vi "configuration UI.vi"() -> ()   [LabVIEW 2013, in "Modbus Module editor node.lvclass"]
doc: "Platypus Framework 1.0.1.65\nNI Systems Engineering - National Instruments"
uses:
  Modbus Module editor node.lvclass
  <vilib>/NI/Configuration Framework/Node/NodeRef.ctl
  <vilib>/NI/Configuration Framework/Node/NISE_CEF_Node.lvclass
  <vilib>/NI/AMC/Message Queue.ctl
  <vilib>/NI/AMC/Message.ctl
  <vilib>/NI/Tools/Keyed Array/KeyedArray.ctl
  <vilib>/NI/Configuration Framework/Node/UserEventRef.ctl
  <vilib>/NI/Configuration Framework/Controls/EventCluster.ctl
  <vilib>/NI/DCAF UI Toolkit/Controls/Configure.ctl
  <vilib>/NI/DCAF UI Toolkit/Controls/Add.ctl
  <vilib>/NI/DCAF UI Toolkit/Controls/Remove.ctl
  <vilib>/NI/DCAF UI Toolkit/Controls/Export.ctl
  module/configuration/modbus class.ctl
  <vilib>/NI/Configuration Framework/Node/NodeChangeEvent.ctl
  <vilib>/NI/DCAF/Tag Editor Core/control module/editor node/channel action event.ctl
  <vilib>/NI/DCAF/Tag Editor Core/control module/editor node/dialog output action.ctl
  <vilib>/NI/Tag Bus Module Framework/channel/TBM channel.lvclass
  <vilib>/NI/Tag Bus/tag/tag descriptor.lvclass
  <vilib>/NI/Configuration Framework/Node/CacheState.ctl
  <vilib>/NI/Configuration Framework/Node/StopEvent.ctl
  <vilib>/NI/Configuration Framework/Node/RefreshUIEvent.ctl
  <vilib>/Utility/miscctls.llb/LVRowAndColumnTypeDef.ctl
  <vilib>/NI/DCAF Table API/Listbox/Multi Column Listbox.lvclass
  <vilib>/NI/DCAF Table API/Table Manager/references.ctl
  <vilib>/NI/DCAF Table API/Listbox/Multi Column Listbox.lvclass/Multi Column Listbox.ctl
  <vilib>/NI/DCAF Table API/Table Manager/Table Manager.lvclass/Table Manager.ctl
  module/configuration/Modbus Module configuration.lvclass
  module/configuration/Modbus Module configuration.lvclass/Modbus Module configuration.ctl
  <vilib>/NI/DCAF/Tag Editor Core/Configuration Editor/Classes/Module editor node/module editor node.lvclass
  module/configuration/modbus mapping behavior.ctl
  module/configuration/Read port (502).vi
  module/configuration/Read baud rate.vi
  module/configuration/Read class.vi
  module/configuration/Read flow control (none).vi
  module/configuration/Read parity (even).vi
  module/configuration/Read serial type.vi
  module/configuration/Read unit ID.vi
  module/configuration/Read VISA resource name.vi
  module/configuration/Read IP address.vi
  module/configuration/Write port (502).vi
  module/configuration/Write baud rate.vi
  module/configuration/Write class.vi
  module/configuration/Write flow control (none).vi
  module/configuration/Write parity (even).vi
  module/configuration/Write serial type.vi
  module/configuration/Write unit ID.vi
  module/configuration/Write VISA resource name.vi
  module/configuration/Write IP address.vi
  module/configuration/Read modbus channels.vi
  <vilib>/NI/DCAF Table API/Listbox/Write Listbox.vi
  <vilib>/NI/DCAF Table API/Table Manager/Write Top VI.vi
  <vilib>/NI/DCAF/Tag Editor Core/Configuration Editor/Classes/Module editor node/Read Module Configuration.vi
  module/configuration/get wire mode.vi
  module/configuration/read force wire mode.vi
  module/configuration/set force wire mode.vi
  module/configuration/set wire mode.vi
  <vilib>/NI/Tag Bus Module Framework/module configuration/TBM module configuration.lvclass
  module/module channel/Modbus Module Channel.lvclass
  <vilib>/NI/Configuration Framework/NISE_CEF_TreeControl.lvlib
  <vilib>/NI/DCAF/Tag Editor Core/control module/editor node/control module editor.lvclass
  <vilib>/NI/Tools/Keyed Array/Tools_KeyedArray.lvlib
  <vilib>/NI/AMC/AMC.lvlib
  <vilib>/NI/DCAF Table API/Table Manager/Table Manager.lvclass
  <vilib>/NI/DCAF UI Toolkit/Controls/DCAF UI Elements.lvlib
panel:
  in  "refresh UI":T1
  in  "stop event":T2
  in  "cache state":T3
  in  "user event out":refnum<user-event>
  in  "node change":T4
  in  "Top Level Tab Control":enum32{"Registers", "Interface", "Export"}(tab)
  in  "settings":T5
  in  "channel":i32(listbox)=1
  in  "Add Button":T6
  in  "Remove Button":T7
  in  "remap":bool
  in  "Settings Tab Control":enum32{"TCP", "Serial"}(tab)
  in  "address":string
  in  "port (502)":u16=502
  in  "set wire mode?":bool
  in  "Wire Mode":T8(ring)
  in  "baud rate":u32
  in  "flow control (none)":u16
  in  "Serial Type":enum16{"RTU", "ASCII"}(ring)
  in  "VISA resource name":refnum<visa-resource-name>
  in  "Parity":enum16{"None", "Odd", "Even", "Mark", "Space"}(ring)
  in  "Unit ID":u8
  in  "Class":T9
  in  "export":T10
  in  "user event":T11
  in  "main queue":T12
  in  "node ref":T13
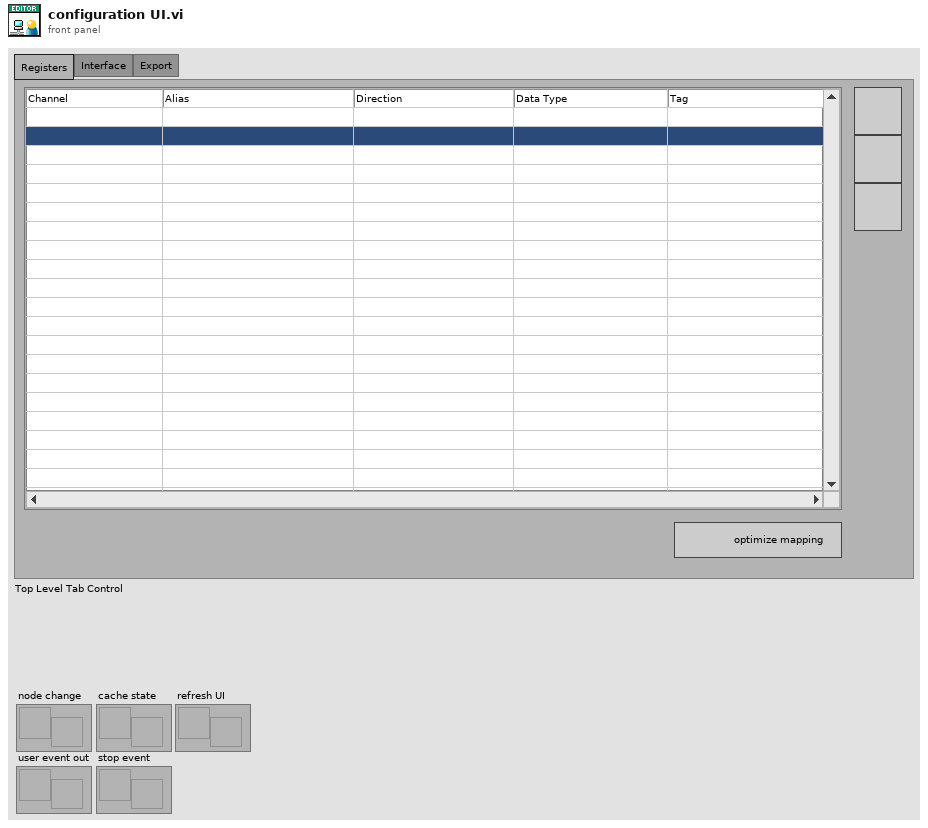
[diagram p1: front panel]
types:
  T1 = typedef "NISE_CEF_Node.lvclass/RefreshUIEvent.ctl" = refnum<user-event>
  T2 = typedef "NISE_CEF_Node.lvclass/StopEvent.ctl" = refnum<user-event>
  T3 = typedef "NISE_CEF_Node.lvclass/CacheState.ctl" = refnum<user-event>
  T4 = typedef "NISE_CEF_Node.lvclass/NodeChangeEvent.ctl" = refnum<user-event>
  T5 = typedef "DCAF UI Elements.lvlib/Configure.ctl" = bool
  T6 = typedef "DCAF UI Elements.lvlib/Add.ctl" = bool
  T7 = typedef "DCAF UI Elements.lvlib/Remove.ctl" = bool
  T8 = enum16{"Unknown", "RS485/Wire4", "RS485/Wire2-EchoDTR", "RS485/Wire2-CtrlDTR", "RS485/Wire2-Auto", "RS232/DTE", "RS232/DCE", "RS232/AUTO"}
  T9 = typedef "Modbus Module configuration.lvclass/modbus class.ctl" = enum16{"TCP master", "TCP slave", "serial master", "serial slave"}
  T10 = typedef "DCAF UI Elements.lvlib/Export.ctl" = bool
  T11 = typedef "NISE_CEF_Node.lvclass/UserEventRef.ctl" = refnum<user-event>
  T12 = typedef "AMC.lvlib/Message Queue.ctl" = refnum<queue>
  T13 = typedef "NISE_CEF_Node.lvclass/NodeRef.ctl" = refnum<data-value>
  T14 = typedef "Table Manager.lvlib/Table Manager.lvclass/references.ctl" = cluster{"stop event":T2, "refresh UI":T1, "cache state":T3, "node change":T4, "user event out":refnum<user-event>, "main queue":T12, "user event":T11}
  T15 = typedef "LVRowAndColumnTypeDef.ctl" = cluster{"Row":i32, "Column":i32}
  T16 = typedef "Table Manager.lvlib/Table Manager.lvclass/object ref.ctl" = cluster{"engine":refnum<data-value>, "Node Ref":refnum<data-value>}
  T17 = typedef "Table Manager.lvlib/Column.lvclass/Column Descriptor.ctl" = cluster{"name":string, "caption":string, "Column Type":T18, "Params":string, "AutoSizeMode":i32, "FillWeight":sgl, "MinWidth":u32, "tooltip":string, "Enum Reference":refnum<vi>, "Channel suffix":string, "Read Only":bool, "Call Back VI":T19, "DT Dependency":i32, "name dependency":i32, "data type":T20}
  T18 = typedef "Table Manager.lvlib/Column.lvclass/Column Type.ctl" = enum16{"String", "Mapping", "Channel Name", "Tag", "Enum", "Data Type", "Numeric"}
  T19 = typedef "Table Manager.lvlib/Table Manager.lvclass/Call Back Ref Type Def.ctl" = refnum<vi>
  T20 = typedef "tag bus.lvlib/tag descriptor.lvclass/Data Type.ctl" = enum16{"Double", "Single", "I64", "I32", "I16", "I8", "U64", "U32", "U16", "U8", "Boolean", "String", "Array of Double", "Array of Single", "Array of I64", "Array of I32", "Array of I16", "Array of I8", "Array of U64", "Array of U32", "Array of U16", "Array of U8", "Array of Boolean", "Array of String"}
  T21 = typedef "Modbus Module configuration.lvclass/modbus mapping behavior.ctl" = enum16{"custom", "optimized"}
  T22 = typedef "Modbus Slave configuration.lvclass/modbus class.ctl" = enum16{"TCP master", "TCP slave", "serial master", "serial slave"}
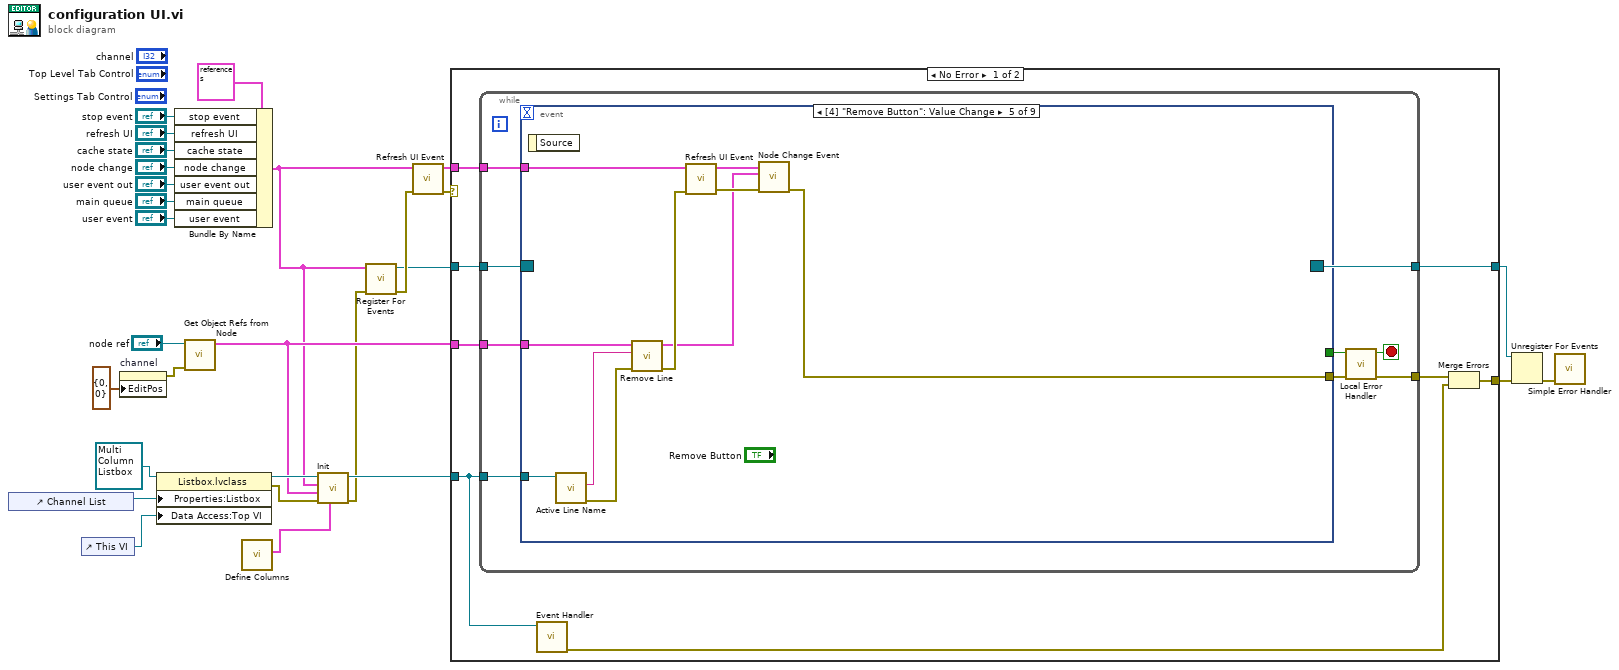
[diagram p0: block diagram]
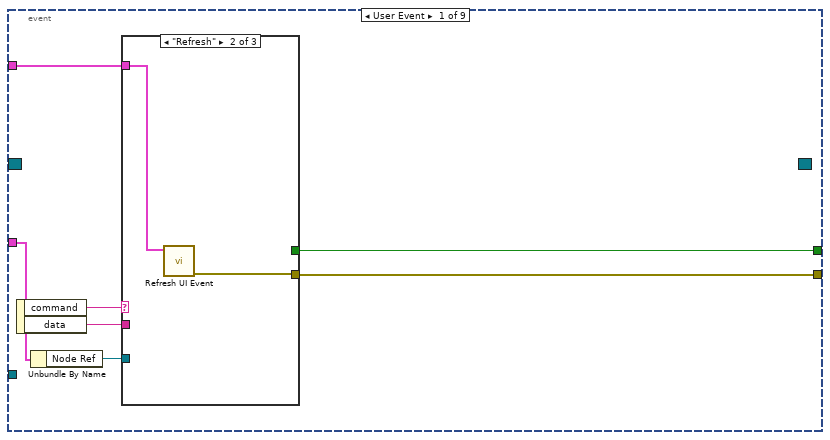
[diagram p2: hidden frame]
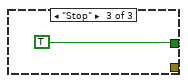
[diagram p4: hidden frame]
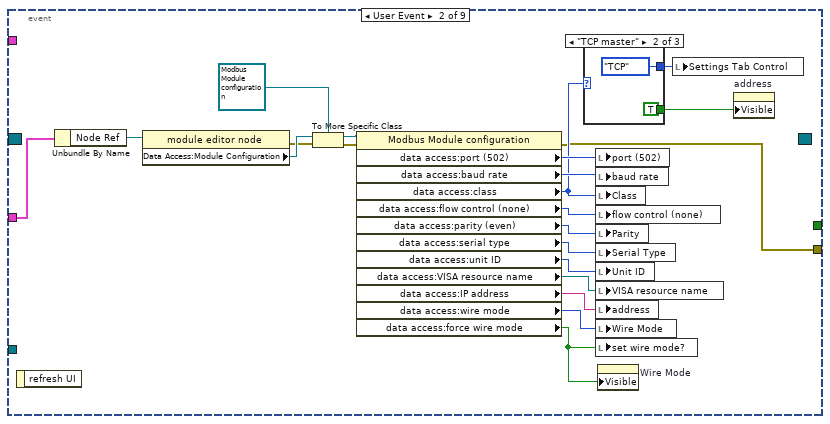
[diagram p5: hidden frame]
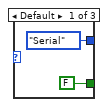
[diagram p6: hidden frame]
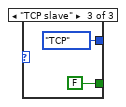
[diagram p7: hidden frame]
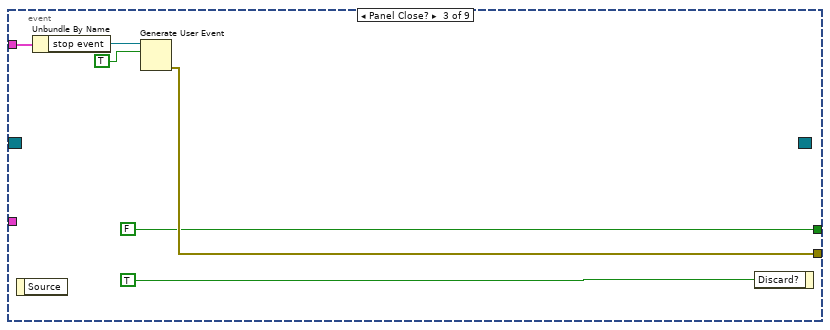
[diagram p8: hidden frame]
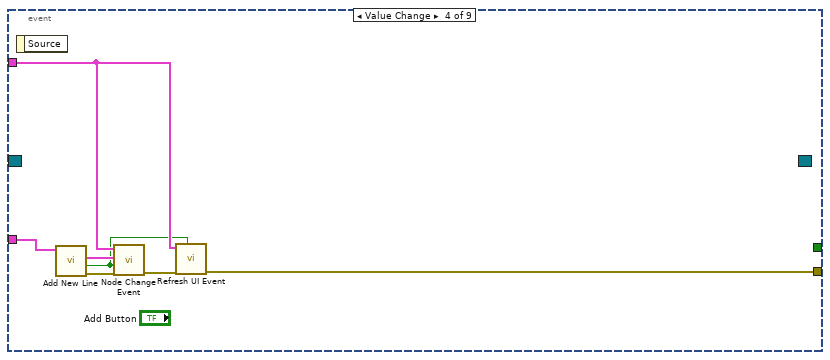
[diagram p9: hidden frame]
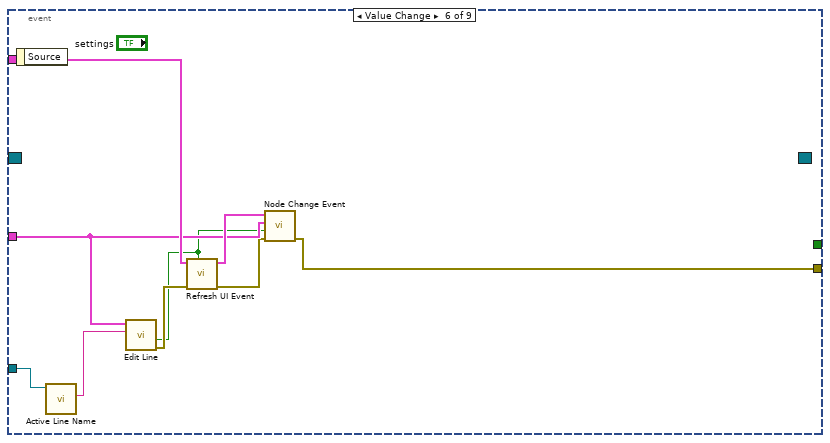
[diagram p10: hidden frame]
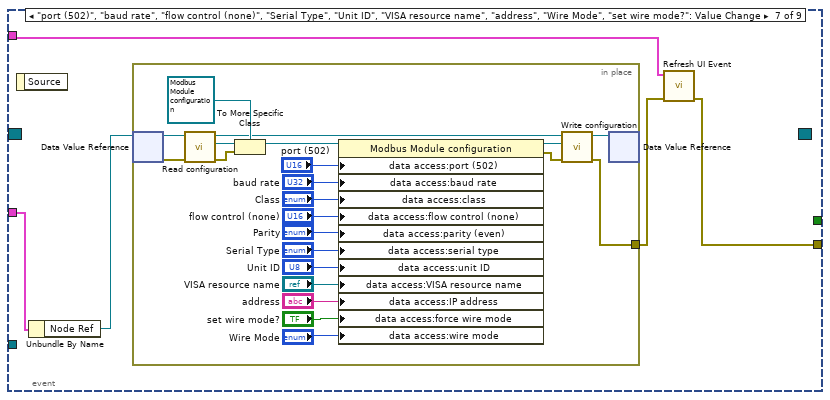
[diagram p11: hidden frame]
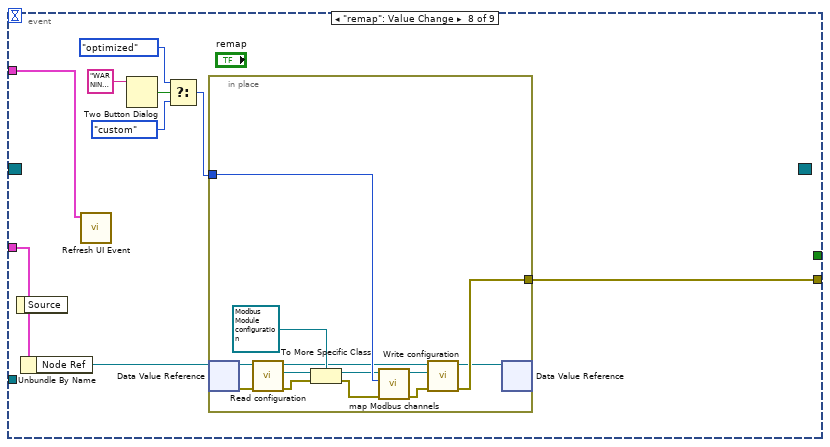
[diagram p12: hidden frame]
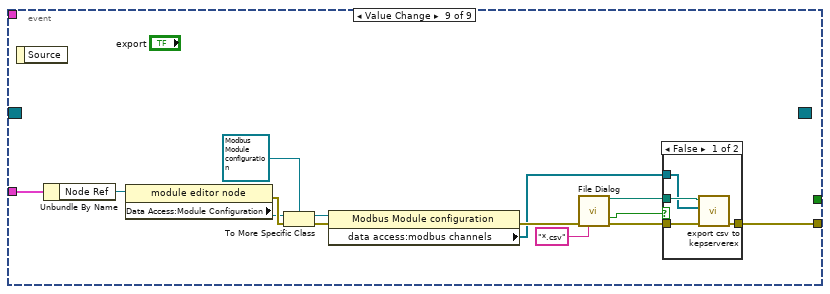
[diagram p13: hidden frame]
diagram:
  n1 = control-ref of="Channel List"() -> (w20:refnum<vi>)
  n2 = control-ref of="This VI"() -> (w21:refnum<vi>)
  n3 = property on="channel" class="MCListbox (strict)"("EditPos"=T15 {"Row"=0, "Column"=0} ("Edit Position")) -> (error out=w13:errorcluster)  [unwired: 2 in, 1 out]
  n4 = property class="Listbox.lvclass"(reference=refnum<class "Multi Column Listbox.lvclass"> refnum ("Multi Column Listbox in"), "Properties:Listbox"=w20, "Data Access:Top VI"=w21) -> (reference out=w22:refnum<class "Multi Column Listbox.lvclass">, error out=w4:errorcluster)  [unwired: 1 in]
  n5 = Bundle By Name(cluster=T14 {"stop event"=refnum, "refresh UI"=refnum, "cache state"=refnum, "node change"=refnum, "user event out"=refnum, "main queue"=refnum, "user event"=refnum} ("References in"), "stop event"="stop event", "refresh UI"="refresh UI", "cache state"="cache state", "node change"="node change", "user event out"="user event out", "main queue"="main queue", "user event"="user event") -> (w3:T14)
  n6 = call "Get Object Refs from Node.vi"("error in (no error)"=w13, "Data Value Reference in"="node ref") -> ("object Refs"=w6:T16)  [unwired: 8 in, 1 out]
  n7 = call "Define Columns.vi"() -> ("Column Definitions"=w1:T17[])  [unwired: 11 in]
  n8 = call-dynamic "Init.vi"("Column Definitions"=w1, "error in (no error)"=w4, "object refs"=w6, "References in"=w3, "Multi Column Listbox in"=w22) -> ("error out"=w2:errorcluster, "Multi Column Listbox out"=w19:refnum<class "Multi Column Listbox.lvclass">)  [unwired: 4 in, 1 out]
  n9 = call "Register For Events.vi"("error in (no error)"=w2, "References in"=w3) -> ("error out"=w16:errorcluster, "Event Registration Refnum"=w15:refnum<event-registration>)  [unwired: 8 in]
  n10 = call "Refresh UI Event.vi"("error in"=w16, "References in"=w3) -> ("error out"=w5:errorcluster, "References out"=w14:T14)  [unwired: 8 in]
  n11 = case shown="No Error" w5 {
    selector: w5 -> [_ w184]
    tunnel: [w36 w183] -> w28
    tunnel: [w29 w184] -> w27
    tunnel: w19 -> [w35 _]
    tunnel: w15 -> [w34 w183]
    tunnel: w14 -> [w33 _]
    tunnel: w6 -> [w32 _]
    frame No Error {
      n12 = while {
        tunnel: [w45] -> w36
        tunnel: [w43] -> w31
        tunnel: w35 -> [w40]
        tunnel: w34 -> [w39]
        tunnel: w33 -> [w38]
        tunnel: w32 -> [w37]
        stop <- w44 stop-if-true
        n13 = event shown="[4] \"Remove Button\": Value Change" {
          selector: w39 -> [_ _ _ _ _ _ _ _ _]
          dyn-events: [_ _ _ _ _ _ _ _ _] -> w45
          timeout: _ -> [_ _ _ _ _ _ _ _ _]
          tunnel: [w52 _ FALSE _ _ _ _ _ _] -> w41
          tunnel: [w49 w59 w87 w90 w99 w106 w115 w142 w173] -> w42
          tunnel: w40 -> [_ _ _ _ w105 w113 _ _ _]
          tunnel: w38 -> [w46 _ w86 w91 w96 w112 w117 w145 _]
          tunnel: w37 -> [w48 w76 _ w95 w102 w110 w119 w144 w165]
          event User Event {
            n14 = event-data() -> ("command"=w51:string, "data"=w50:string)  [unwired: 1 in]
            n15 = Unbundle By Name(w48) -> ("Node Ref"=w47:refnum<data-value>)
            n16 = case shown="\"Refresh\"" w51 {
              tunnel: [_ _ TRUE] -> w52
              tunnel: w50 -> [_ _ _]
              tunnel: [_ w53 _] -> w49
              tunnel: w47 -> [_ _ _]
              tunnel: w46 -> [_ w54 _]
              frame Default {
              }
              frame "Refresh" {
                n17 = call "Refresh UI Event.vi"("References in"=w54) -> ("error out"=w53:errorcluster)  [unwired: 9 in, 1 out]
              }
              frame "Stop" {
              }
            }
          }
          event User Event {
            n18 = event-data() -> ()  [unwired: 1 in, 1 out]
            n19 = Unbundle By Name(w76) -> ("Node Ref"=w75:refnum<data-value>)
            n20 = property class="module editor node"(reference=w75) -> (error out=w61:errorcluster, "Data Access:Module Configuration"=w73:refnum<class "TBM module configuration.lvclass">)  [unwired: 1 in, 1 out]
            n21 = To More Specific Class(target class=refnum<class "Modbus Module configuration.lvclass"> refnum ("tag bus configurable plugin module configuration"), reference=w73, error in=w61) -> (specific class reference=w64:refnum<class "Modbus Module configuration.lvclass">, error out=w60:errorcluster)
            n22 = property class="Modbus Module configuration"(reference=w64, error in=w60) -> (error out=w59:errorcluster, "data access:port (502)"=w68:u16, "data access:baud rate"=w65:u32, "data access:class"=w63:T22, "data access:flow control (none)"=w69:u16, "data access:parity (even)"=w70:u16, "data access:serial type"=w71:enum16{"RTU", "ASCII"}, "data access:unit ID"=w67:u8, "data access:VISA resource name"=w66:refnum<visa-resource-name>, "data access:IP address"=w72:string, "data access:wire mode"=w57:i16, "data access:force wire mode"=w58:bool)  [unwired: 1 out]
            n23 = case shown="\"TCP master\"" w63 {
              tunnel: [enum32{"TCP", "Serial"}."Serial" ("Settings Tab Control") enum32{"TCP", "Serial"}."TCP" ("Settings Tab Control") enum32{"TCP", "Serial"}."TCP" ("Settings Tab Control")] -> w62
              tunnel: [FALSE TRUE FALSE] -> w56
              frame Default {
              }
              frame "TCP master" {
              }
              frame "TCP slave" {
              }
            }
            n24 = local write "port (502)"(w68) -> ()
            n25 = local write "baud rate"(w65) -> ()
            n26 = local write "Class"(w63) -> ()
            n27 = local write "flow control (none)"(w69) -> ()
            n28 = local write "Parity"(w70) -> ()
            n29 = local write "Serial Type"(w71) -> ()
            n30 = local write "Unit ID"(w67) -> ()
            n31 = local write "VISA resource name"(w66) -> ()
            n32 = local write "address"(w72) -> ()
            n33 = local write "Wire Mode"(w57) -> ()
            n34 = local write "set wire mode?"(w58) -> ()
            n35 = property on="Wire Mode" class="Enum (strict)"("Visible"=w58) -> ()  [unwired: 2 in, 2 out]
            n36 = local write "Settings Tab Control"(w62) -> ()
            n37 = property on="address" class="Str"("Visible"=w56) -> ()  [unwired: 2 in, 2 out]
          }
          event Panel Close? {
            n38 = event-data() -> ()  [unwired: 1 in, 1 out]
            n39 = Unbundle By Name(w86) -> ("stop event"=w85:T2)
            n40 = Generate User Event(user event=w85, event data cluster=TRUE ("event data")) -> (error out=w87:errorcluster)  [unwired: 2 in, 1 out]
            n41 = event-data("Discard?"=TRUE) -> ()  [unwired: 1 in, 1 out]
          }
          event Value Change {
            n42 = event-data() -> ()  [unwired: 1 in, 1 out]
            n43 = call "Add New Line.vi"("Object Refs"=w95) -> ("error out"=w93:errorcluster, "Success"=w89:bool, "Object Refs  out"=w94:T16)  [unwired: 8 in]
            n44 = call "Node Change Event.vi"("error in"=w93, "Send"=w89, "object Refs"=w94, "References in"=w91) -> ("error out"=w92:errorcluster)  [unwired: 7 in]
            n45 = call "Refresh UI Event.vi"("Refresh"=w89, "error in"=w92, "References in"=w91) -> ("error out"=w90:errorcluster)  [unwired: 7 in, 1 out]
          }
          event Value Change {
            n46 = event-data() -> ()  [unwired: 1 in, 1 out]
            n47 = call-dynamic "Active Line Name.vi"("Multi Column Listbox in"=w105) -> ("error out"=w103:errorcluster, "Active Line Name"=w104:string)  [unwired: 8 in, 1 out]
            n48 = call "Remove Line.vi"("error in (no error)"=w103, "Active Line Name"=w104, "object Refs in"=w102) -> ("error out"=w98:errorcluster, "object Refs out"=w97:T16)  [unwired: 7 in]
            n49 = call "Refresh UI Event.vi"("error in"=w98, "References in"=w96) -> ("error out"=w100:errorcluster, "References out"=w101:T14)  [unwired: 8 in]
            n50 = call "Node Change Event.vi"("error in"=w100, "object Refs"=w97, "References in"=w101) -> ("error out"=w99:errorcluster)  [unwired: 8 in]
          }
          event Value Change {
            n51 = event-data() -> ()  [unwired: 1 in, 1 out]
            n52 = call-dynamic "Active Line Name.vi"("Multi Column Listbox in"=w113) -> ("Active Line Name"=w114:string)  [unwired: 8 in, 2 out]
            n53 = call "Edit Line.vi"("Line Name"=w114, "object Refs"=w110) -> ("error out"=w109:errorcluster, "Change"=w107:bool)  [unwired: 8 in]
            n54 = call "Refresh UI Event.vi"("Refresh"=w107, "error in"=w109, "References in"=w112) -> ("error out"=w108:errorcluster, "References out"=w111:T14)  [unwired: 7 in]
            n55 = call "Node Change Event.vi"("error in"=w108, "Send"=w107, "object Refs"=w110, "References in"=w111) -> ("error out"=w106:errorcluster)  [unwired: 7 in]
          }
          event "port (502)", "baud rate", "flow control (none)", "Serial Type", "Unit ID", "VISA resource name", "address", "Wire Mode", "set wire mode?": Value Change {
            n56 = event-data() -> ()  [unwired: 1 in, 1 out]
            n57 = Unbundle By Name(w119) -> ("Node Ref"=w118:refnum<data-value>)
            n58 = in-place {
              in-place-border: [w122] -> w116
              n59 = in-place-dvr #1(w118) -> (w130:refnum<class "module editor node.lvclass">, w120:errorcluster)
              n60 = call-dynamic "Read configuration.vi"("error in"=w120, "NISE_CEF_serializable node in"=w130) -> ("error out"=w121:errorcluster, "configuration"=w128:refnum<class "NISE_CEF_serializable configuration.lvclass">, "NISE_CEF_serializable node out"=w126:refnum<class "module editor node.lvclass">)  [unwired: 7 in]
              n61 = To More Specific Class(target class=refnum<class "Modbus Module configuration.lvclass"> refnum ("Modbus Module configuration"), reference=w128, error in=w121) -> (specific class reference=w127:refnum<class "Modbus Module configuration.lvclass">)  [unwired: 1 out]
              n62 = property class="Modbus Module configuration"(reference=w127, "data access:port (502)"="port (502)", "data access:baud rate"="baud rate", "data access:class"="Class", "data access:flow control (none)"="flow control (none)", "data access:parity (even)"="Parity", "data access:serial type"="Serial Type", "data access:unit ID"="Unit ID", "data access:VISA resource name"="VISA resource name", "data access:IP address"="address", "data access:force wire mode"="set wire mode?", "data access:wire mode"="Wire Mode") -> (reference out=w125:refnum<class "Modbus Module configuration.lvclass">, error out=w123:errorcluster)  [unwired: 1 in]
              n63 = call-dynamic "Write configuration.vi"("error in"=w123, "configuration"=w125, "NISE_CEF_serializable node in"=w126) -> ("error out"=w122:errorcluster, "NISE_CEF_serializable node out"=w124:refnum<class "module editor node.lvclass">)  [unwired: 7 in]
              n64 = in-place-dvr #1(w124) -> ()  [unwired: 2 out]
            }
            n65 = call "Refresh UI Event.vi"("error in"=w116, "References in"=w117) -> ("error out"=w115:errorcluster)  [unwired: 8 in, 1 out]
          }
          event "remap": Value Change {
            n66 = event-data() -> ()  [unwired: 1 in, 1 out]
            n67 = Unbundle By Name(w144) -> ("Node Ref"=w143:refnum<data-value>)
            n68 = call "Refresh UI Event.vi"("References in"=w145) -> ()  [unwired: 9 in, 2 out]
            n69 = Two Button Dialog(message="WARNING! This will reorder register mappings and cannot be undone. Press \"OK\" to proceed or \"Cancel\" to keep current mappings.") -> (T button?=w149:bool)  [unwired: 2 in]
            n70 = Select(t=modbus_mapping_behavior."optimized" ("Mapping"), s=w149, f=modbus_mapping_behavior."custom" ("Mapping")) -> (s? t:f=w146:T21)
            n71 = in-place {
              in-place-border: w146 -> [w163]
              in-place-border: [w155] -> w142
              n72 = in-place-dvr #2(w143) -> (w162:refnum<class "module editor node.lvclass">, w161:errorcluster)
              n73 = call-dynamic "Read configuration.vi"("error in"=w161, "NISE_CEF_serializable node in"=w162) -> ("error out"=w157:errorcluster, "configuration"=w153:refnum<class "NISE_CEF_serializable configuration.lvclass">, "NISE_CEF_serializable node out"=w151:refnum<class "module editor node.lvclass">)  [unwired: 7 in]
              n74 = To More Specific Class(target class=refnum<class "Modbus Module configuration.lvclass"> refnum ("Modbus Slave configuration in"), reference=w153, error in=w157) -> (specific class reference=w159:refnum<class "Modbus Module configuration.lvclass">, error out=w158:errorcluster)
              n75 = call "map Modbus channels.vi"("error in"=w158, "mapping"=w163, "Modbus Slave configuration in"=w159) -> ("error out"=w156:errorcluster, "Modbus Slave configuration out"=w152:refnum<class "Modbus Module configuration.lvclass">)  [unwired: 7 in]
              n76 = call-dynamic "Write configuration.vi"("error in"=w156, "configuration"=w152, "NISE_CEF_serializable node in"=w151) -> ("error out"=w155:errorcluster, "NISE_CEF_serializable node out"=w154:refnum<class "module editor node.lvclass">)  [unwired: 7 in]
              n77 = in-place-dvr #2(w154) -> ()  [unwired: 2 out]
            }
          }
          event Value Change {
            n78 = event-data() -> ()  [unwired: 1 in, 1 out]
            n79 = Unbundle By Name(w165) -> ("Node Ref"=w164:refnum<data-value>)
            n80 = property class="module editor node"(reference=w164) -> (error out=w172:errorcluster, "Data Access:Module Configuration"=w169:refnum<class "TBM module configuration.lvclass">)  [unwired: 1 in, 1 out]
            n81 = To More Specific Class(target class=refnum<class "Modbus Module configuration.lvclass"> refnum ("tag bus configurable plugin module configuration"), reference=w169, error in=w172) -> (specific class reference=w168:refnum<class "Modbus Module configuration.lvclass">, error out=w170:errorcluster)
            n82 = property class="Modbus Module configuration"(reference=w168, error in=w170) -> (error out=w171:errorcluster, "data access:modbus channels"=w166:refnum<class "Modbus Module Channel.lvclass">[])  [unwired: 1 out]
            n83 = call "File Dialog"("error in"=w171, "pattern (all files)"="*.csv") -> ("selected path"=w177:path, "cancelled"=w174:bool, "error out"=w175:errorcluster)  [unwired: 10 in, 1 out]
            n84 = case shown="False" w174 {
              tunnel: w177 -> [w179 _]
              tunnel: w175 -> [w180 w182]
              tunnel: [w181 w182] -> w173
              tunnel: w166 -> [w178 _]
              frame False {
                n85 = call "export csv to kepserverex.vi"("error in"=w180, "modbus channels"=w178, "selected path"=w179) -> ("error out"=w181:errorcluster)  [unwired: 8 in]
              }
              frame True {
              }
            }
          }
        }
        n86 = call "Local Error Handler.vi"("error in (no error)"=w42, "Boolean in"=w41) -> ("error out"=w43:errorcluster, "Boolean out"=w44:bool)  [unwired: 8 in]
      }
      n87 = call-dynamic "Event Handler.vi"("Listbox in"=w35) -> ("error out"=w30:errorcluster)  [unwired: 9 in, 1 out]
      n88 = Merge Errors(w31, w30) -> (w29:errorcluster)
    }
    frame Error {
    }
  }
  n89 = Unregister For Events(event registration refnum=w28, error in=w27) -> (error out=w25:errorcluster)
  n90 = call <vilib>:"Simple Error Handler.vi"("error in (no error)"=w25) -> ()  [unwired: 4 in, 5 out]
